vi "Find Center Setup.vi"(0 "Carrier Tray":T2, 1 "Tray Number":dbl format="%#_13g", 2 "Position":i32, 3 "Type of Hexaboard":T1) -> (7 "Assembly Tray Out":T2)   [LabVIEW 2021, in "Assembly Tray.lvclass"]
uses:
  Assembly Tray.lvclass
  Find Tray.ctl
  Routine/TypeOfHexaboard.ctl
  Routine/Routine.lvclass
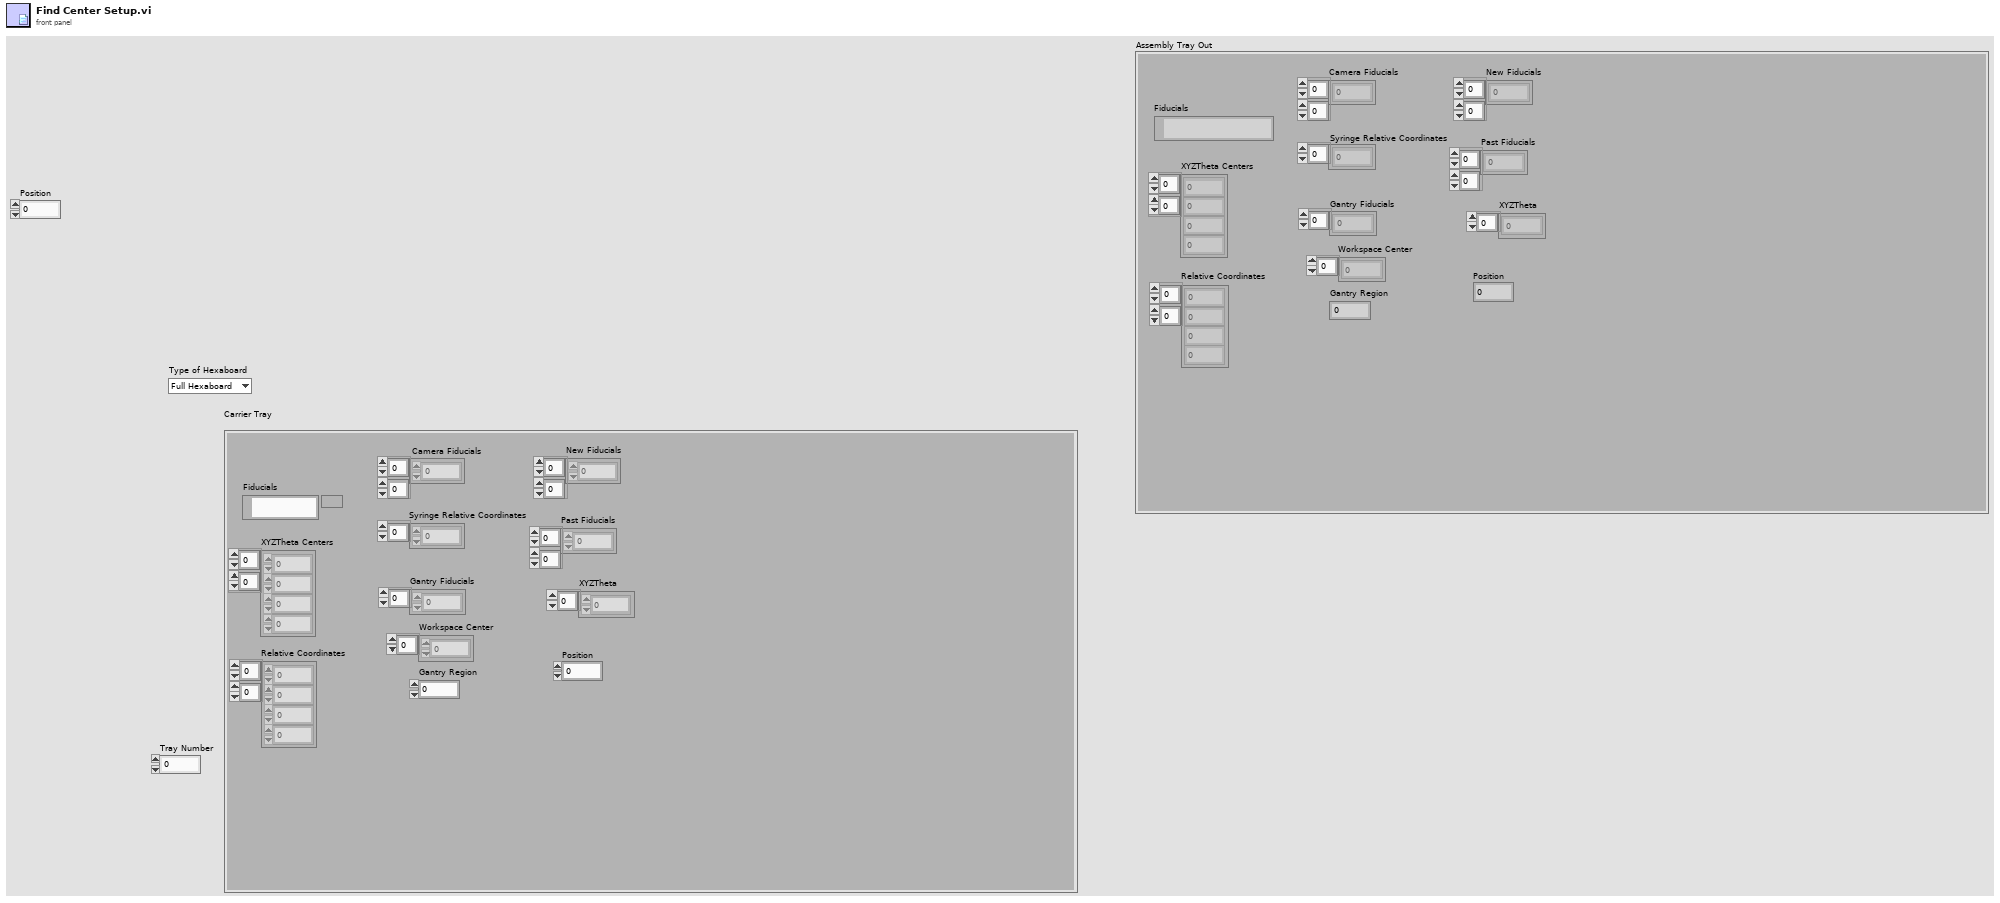
[diagram p1: front panel]
types:
  T1 = typedef "Routine.lvclass/TypeOfHexaboard.ctl" = enum16{"Full Hexaboard", "Right Partial PCB", "Right Partial Sensor", "Al Dummy Right Partial Sensor"}
  T2 = typedef "Assembly Tray.lvclass/Find Tray.ctl" = cluster{"Gantry Fiducials":dbl[], "Relative Coordinates":dbl[][], "Camera Fiducials":dbl[][], "XYZTheta Centers":dbl[][], "Workspace Center":dbl[], "Syringe Relative Coordinates":dbl[], "Gantry Region":dbl, "Fiducials":path, "New Fiducials":dbl[][], "Past Fiducials":dbl[][], "XYZTheta":dbl[], "Position":dbl}
  T3 = typedef "File Paths.ctl" = cluster{"Glue Pattern Folder":path, "Carrier Tray Folder":path, "Pick Up Tool Fixture Folder":path, "Components Folder":path, "Bellows Tool Offset.txt":path, "Pick Up Tool Offset.txt":path, "Dispense Tip Offset.txt":path, "Log Files":path, "Gantry Assembly Map.txt":path, "Syringe and offset map.txt":path}
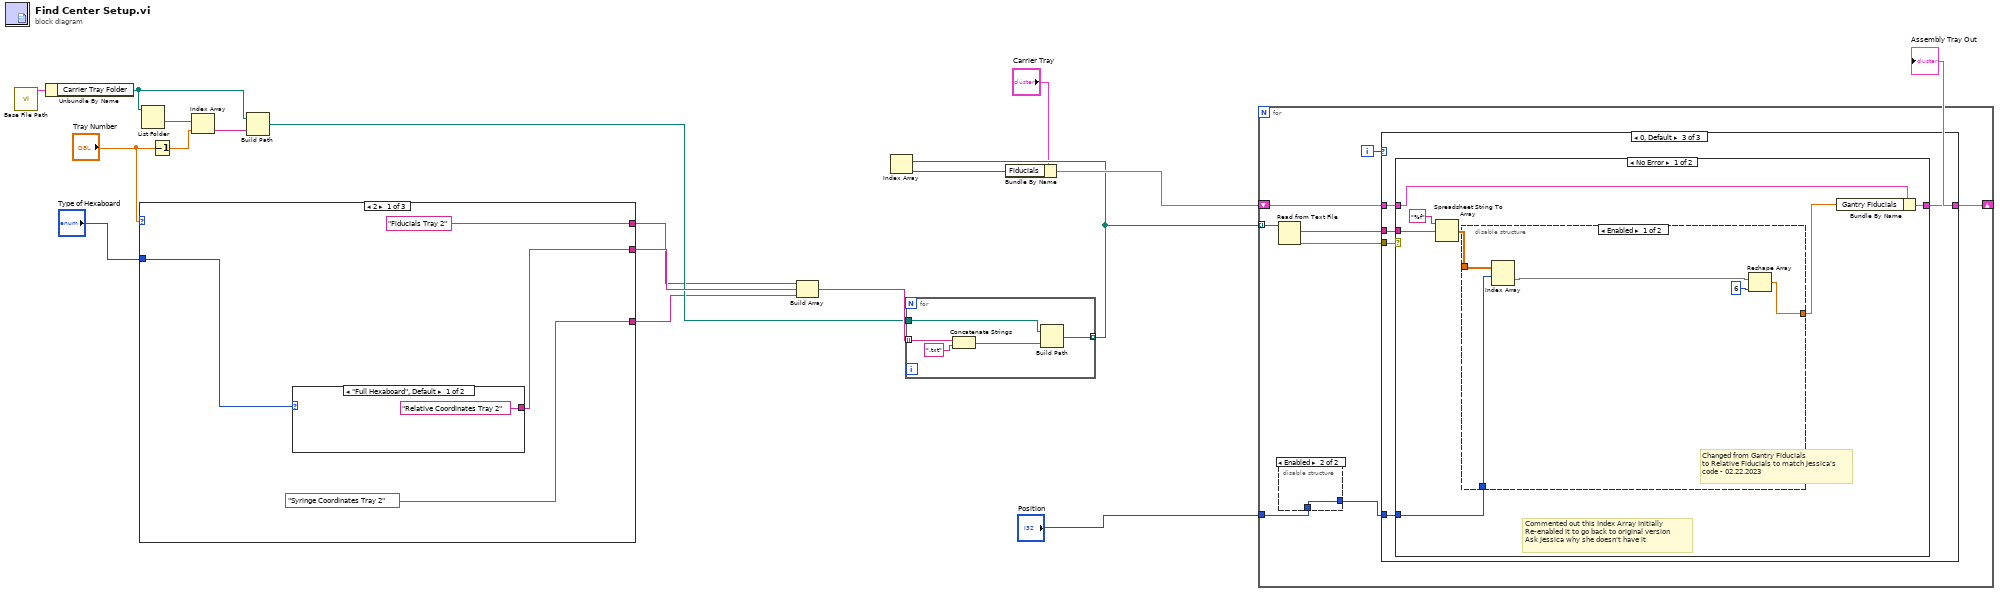
[diagram p0: block diagram]
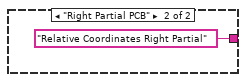
[diagram p2: hidden frame]
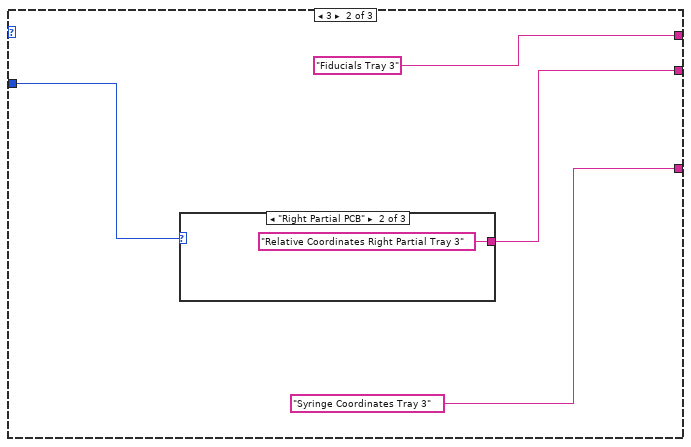
[diagram p3: hidden frame]
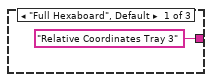
[diagram p4: hidden frame]
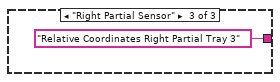
[diagram p5: hidden frame]
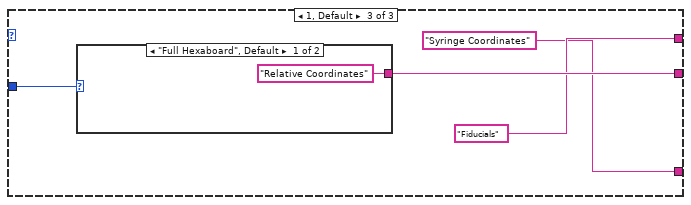
[diagram p6: hidden frame]
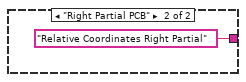
[diagram p7: hidden frame]
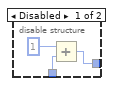
[diagram p8: hidden frame]
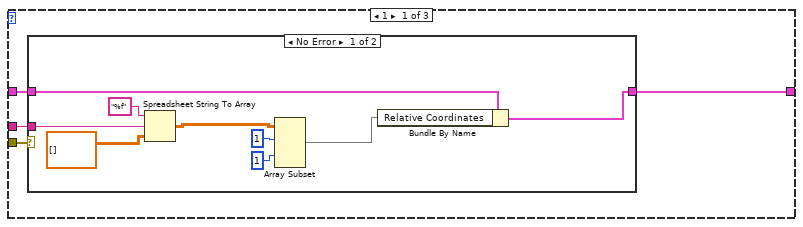
[diagram p9: hidden frame]
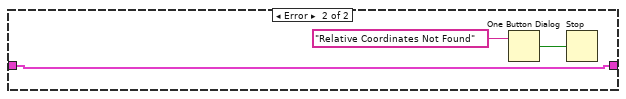
[diagram p10: hidden frame]
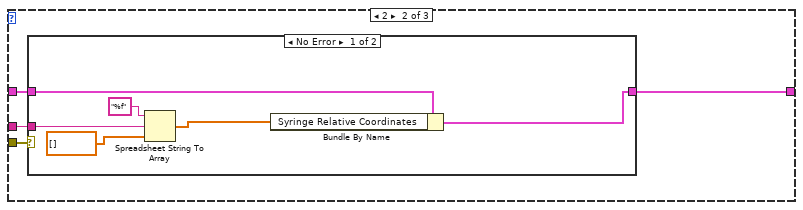
[diagram p11: hidden frame]
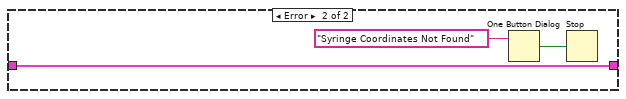
[diagram p12: hidden frame]
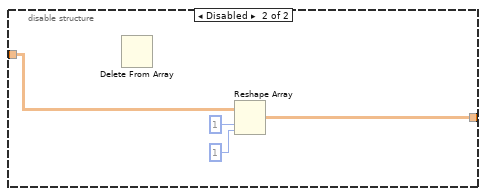
[diagram p13: hidden frame]
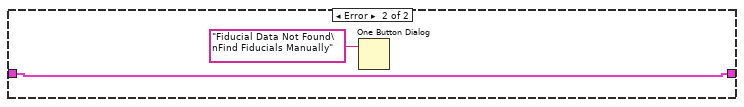
[diagram p14: hidden frame]
diagram:
  n1 = call "Base File Path.vi"() -> ("Paths Out"=w13:T3)  [unwired: 11 in]
  n2 = Unbundle By Name(w13) -> ("Carrier Tray Folder"=w5:path)
  n3 = case shown="2" "Tray Number" {
    tunnel: [w21 w27 w35] -> w8
    tunnel: "Type of Hexaboard" -> [w22 w28 w34]
    tunnel: ["Fiducials Tray 2" ("format string") "Fiducials Tray 3" ("format string") "Fiducials" ("format string")] -> w3
    tunnel: ["Syringe Coordinates Tray 2" ("element") "Syringe Coordinates Tray 3" ("element") "Syringe Coordinates" ("element")] -> w2
    frame 2 {
      n4 = case shown="\"Full Hexaboard\", Default" w22 {
        tunnel: ["Relative Coordinates Tray 2" ("format string") "Relative Coordinates Right Partial" ("format string")] -> w21
        frame "Full Hexaboard", Default {
        }
        frame "Right Partial PCB" {
        }
      }
    }
    frame 3 {
      n5 = case shown="\"Right Partial PCB\"" w28 {
        tunnel: ["Relative Coordinates Tray 3" ("format string") "Relative Coordinates Right Partial Tray 3" ("format string") "Relative Coordinates Right Partial Tray 3" ("format string")] -> w27
        frame "Full Hexaboard", Default {
        }
        frame "Right Partial PCB" {
        }
        frame "Right Partial Sensor" {
        }
      }
    }
    frame 1, Default {
      n6 = case shown="\"Full Hexaboard\", Default" w34 {
        tunnel: ["Relative Coordinates" ("format string") "Relative Coordinates Right Partial" ("format string")] -> w35
        frame "Full Hexaboard", Default {
        }
        frame "Right Partial PCB" {
        }
      }
    }
  }
  n7 = List Folder(path=w5) -> (folder names=w15:string[])  [unwired: 3 in, 3 out]
  n8 = Decrement(x="Tray Number") -> (x-1=w11:dbl)
  n9 = Index Array "Index Array"(array=w15, index=w11) -> (element=w14:string)
  n10 = Build Path(base path=w5, name or relative path=w14) -> (appended path=w6:path)
  n11 = Build Array(w3, w8, w2) -> (w16:string[])
  n12 = for {
    tunnel: w16 -> [w41] mode=indexing
    tunnel: w6 -> [w42]
    tunnel: [w38] -> w7 mode=indexing
    n13 = Concatenate Strings "Concatenate Strings"(w41, ".txt" ("string")) -> (w39:string)
    n14 = Build Path(base path=w42, name or relative path=w39) -> (appended path=w38:path)
  }
  n15 = Index Array "Index Array"(array=w7) -> (element=w17:path)  [unwired: 1 in]
  n16 = Bundle By Name "Bundle By Name"(cluster="Carrier Tray", "Fiducials"=w17) -> (w18:T2)
  n17 = for {
    tunnel: w7 -> [w49] mode=indexing
    shift-right: [w45] -> w12
    shift-left: w18 -> [w46]
    tunnel: "Position" -> [w44]
    i -> [w47]
    n18 = Read from Text File(file (use dialog)=w49) -> (text=w50:string, error out=w48:errorcluster)  [unwired: 3 in, 2 out]
    n19 = disable-structure shown="Enabled" {
      disable-tunnel: w44 -> [w52 w54]
      disable-tunnel: [w51 w54] -> w43
      frame Disabled {
        n20 = Add(x=1, y=w52) -> (x+y=w51:i32)
      }
      frame Enabled {
      }
    }
    n21 = case shown="0, Default" w47 {
      tunnel: w50 -> [w57 w72 w88]
      tunnel: w48 -> [w58 w73 w87]
      tunnel: w46 -> [w56 w74 w86]
      tunnel: [w55 w71 w85] -> w45
      tunnel: w43 -> [_ _ w84]
      frame 1 {
        n22 = case shown="No Error" w58 {
          tunnel: w57 -> [w65 _]
          tunnel: [w63 w68] -> w55
          tunnel: w56 -> [w64 w68]
          frame No Error {
            n23 = Spreadsheet String To Array(format string="%f", spreadsheet string=w65, array type (2D Dbl)=dbl[][] []) -> (array=w62:dbl[][])  [unwired: 1 in]
            n24 = Array Subset(array=w62, index (row)=1 ("length"), index (col)=1 ("index (row)")) -> (w61:dbl[][])  [unwired: 2 in]
            n25 = Bundle By Name(cluster=w64, "Relative Coordinates"=w61) -> (w63:T2)
          }
          frame Error {
            n26 = One Button Dialog(message="Relative Coordinates Not Found") -> (true=w69:bool)  [unwired: 1 in]
            n27 = Stop(stop? (T)=w69) -> ()
          }
        }
      }
      frame 2 {
        n28 = case shown="No Error" w73 {
          tunnel: w72 -> [w78 _]
          tunnel: [w76 w81] -> w71
          tunnel: w74 -> [w77 w81]
          frame No Error {
            n29 = Spreadsheet String To Array(format string="%f", spreadsheet string=w78, array type (2D Dbl)=dbl[] []) -> (array=w75:dbl[])  [unwired: 1 in]
            n30 = Bundle By Name(cluster=w77, "Syringe Relative Coordinates"=w75) -> (w76:T2)
          }
          frame Error {
            n31 = One Button Dialog(message="Syringe Coordinates Not Found") -> (true=w82:bool)  [unwired: 1 in]
            n32 = Stop(stop? (T)=w82) -> ()
          }
        }
      }
      frame 0, Default {
        n33 = case shown="No Error" w87 {
          tunnel: w88 -> [w94 _]
          tunnel: w86 -> [w92 w105]
          tunnel: [w93 w105] -> w85
          tunnel: w84 -> [w89 _]
          frame No Error {
            # "Commented out this Index Array Initially\nRe-enabled it to go back to original version\nAsk Jessica why she doesn't have it"
            # "Changed from Gantry Fiducials\nto Relative Fiducials to match Jessica's \ncode - 02.22.2023"
            n34 = Spreadsheet String To Array(format string="%f", spreadsheet string=w94) -> (array=w90:dbl[][])  [unwired: 2 in]
            n35 = disable-structure shown="Enabled" {
              disable-tunnel: [w100 w101] -> w91
              disable-tunnel: w90 -> [w99 w104]
              disable-tunnel: w89 -> [w96 _]
              frame Enabled {
                n36 = Index Array "Index Array"(array=w99, index (row)=w96) -> (element=w98:dbl[])  [unwired: 1 in]
                n37 = Reshape Array "Reshape Array"(w98, 6 ("dimension size")) -> (w100:dbl[])
              }
              frame Disabled {
                n38 = Delete From Array "Delete From Array"() -> ()  [unwired: 3 in, 2 out]
                n39 = Reshape Array "Reshape Array"(w104, 1 ("dimension size"), 1 ("dimension size")) -> (w101:dbl[][])
              }
            }
            n40 = Bundle By Name "Bundle By Name"(cluster=w92, "Gantry Fiducials"=w91) -> (w93:T2)
          }
          frame Error {
            n41 = One Button Dialog(message="Fiducial Data Not Found\nFind Fiducials Manually") -> ()  [unwired: 1 in, 1 out]
          }
        }
      }
    }
  }
  "Assembly Tray Out" <- w12
